vi "Run.vi"(8 "error in (no error)":errorcluster, 10 "Project Path":string, 11 "TestRunner in":refnum<class "TestRunner.lvclass">) -> (0 "error out":errorcluster, 3 "TestRunner out":refnum<class "TestRunner.lvclass">)   [LabVIEW 2019, in "TestRunner.lvlib" / "TestRunner.lvclass"]
uses:
  TestRunner.lvclass
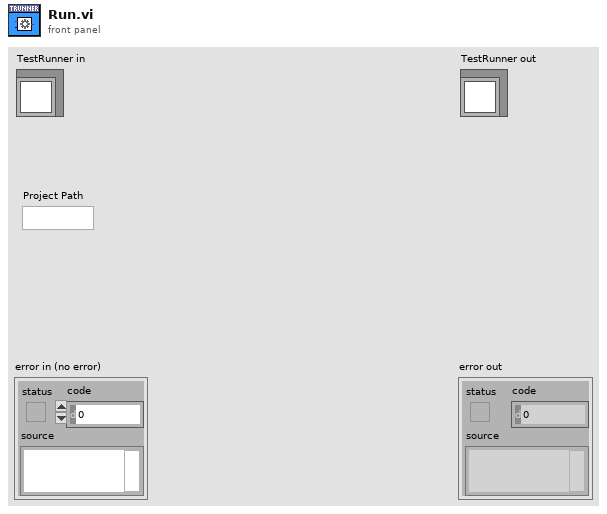
[diagram p1: front panel]
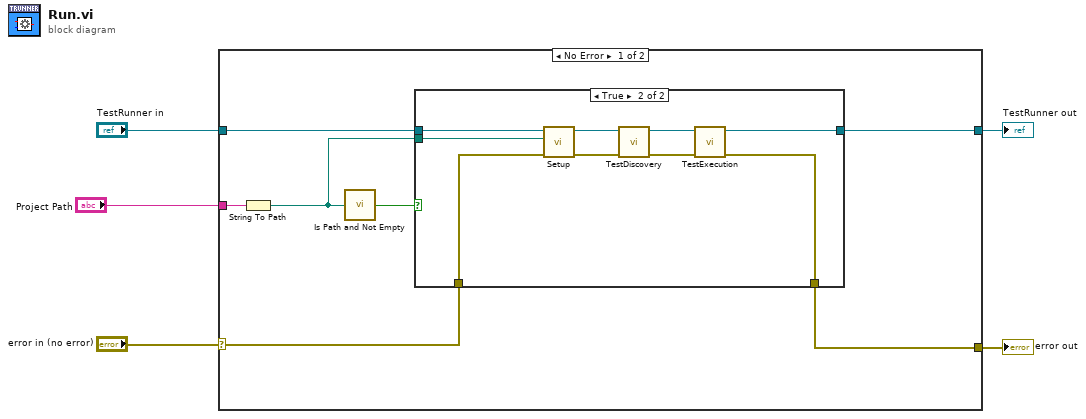
[diagram p0: block diagram]
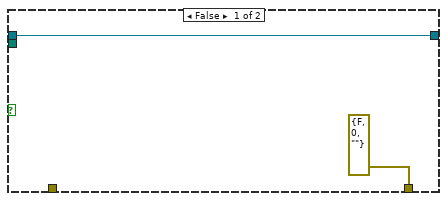
[diagram p2: hidden frame]
diagram:
  n1 = case shown="No Error" "error in (no error)" {
    selector: "error in (no error)" -> [w8 w25]
    tunnel: [w7 w25] -> w4
    tunnel: [w9 w24] -> w2
    tunnel: "TestRunner in" -> [w12 w24]
    tunnel: "Project Path" -> [w11 _]
    frame No Error {
      n2 = String To Path(string=w11) -> (path=w10:path)
      n3 = call <vilib>:"Is Path and Not Empty.vi"("path"=w10) -> ("Is Path and Not Empty?"=w6:bool)  [unwired: 4 in]
      n4 = case shown="True" w6 {
        tunnel: w12 -> [w14 w18]
        tunnel: w10 -> [_ w17]
        tunnel: [w14 w21] -> w9
        tunnel: w8 -> [_ w16]
        tunnel: [errorcluster {"status"=FALSE, "code"=0, "source"=""} ("error out") w20] -> w7
        frame False {
        }
        frame True {
          n5 = call-dynamic "Setup.vi"("error in (no error)"=w16, "Libray Path"=w17, "TestRunner in"=w18) -> ("error out"=w15:errorcluster, "TestRunner out"=w19:refnum<class "TestRunner.lvclass">)  [unwired: 7 in]
          n6 = call-dynamic "TestDiscovery.vi"("error in (no error)"=w15, "TestRunner in"=w19) -> ("error out"=w22:errorcluster, "TestRunner out"=w23:refnum<class "TestRunner.lvclass">)  [unwired: 8 in]
          n7 = call-dynamic "TestExecution.vi"("error in (no error)"=w22, "TestRunner in"=w23) -> ("error out"=w20:errorcluster, "TestRunner out"=w21:refnum<class "TestRunner.lvclass">)  [unwired: 8 in]
        }
      }
    }
    frame Error {
    }
  }
  "error out" <- w4
  "TestRunner out" <- w2
